vi "Configure Network Gateway.vi"(8 "error in (no error)":errorcluster, 10 "Network Gateway (\"\")":string, 11 "VISA resource name":refnum<visa-resource-name>) -> (0 "error out":errorcluster, 3 "VISA resource name out":refnum<visa-resource-name>)   [LabVIEW 2015, in "Rohde&Schwarz CMXP Base.lvlib"]
doc: "Manually defines IPv4 addresses of default gateways. A query returns the currently defined addresses, irrespective of whether they have been specified manually or via DHCP.\n\nAttribute:\nRSCMXPBASE_ATTR_CONFIGURE_NETWORK_GATEWAY\n\nRemote-control command:\nSYSTem:COMMunicate:NET:GATeway"
uses:
  <instrlib>/Rohde&Schwarz CMXP Base/Rohde&Schwarz CMXP Base.lvlib
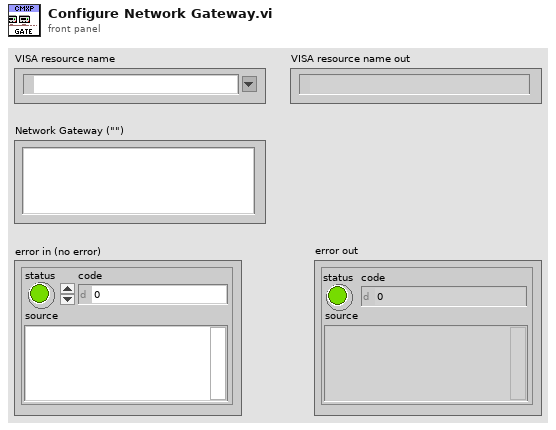
[diagram p1: front panel]
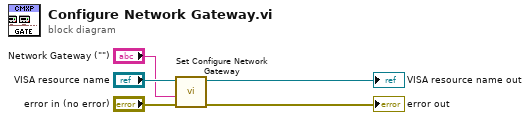
[diagram p0: block diagram]
diagram:
  n1 = call "Set Configure Network Gateway"("error in (no error)"="error in (no error)", "Configure Network Gateway ()"="Network Gateway (\"\")", "instrument handle"="VISA resource name") -> ("error out"=→"error out":errorcluster, "instrument handle out"=→"VISA resource name out":refnum<visa-resource-name>)  [unwired: 7 in]
